vi "GetEdgeMenu.vi"(0 "reference":refnum<class "ClassRelationshipEdge.lvclass">, 5 "error in (no error)":errorcluster) -> (14 "reference out":refnum<class "ClassRelationshipEdge.lvclass">, 15 "MenuOptions":string[](array[string]), 19 "error out":errorcluster)   [LabVIEW 2020, in "ClassRelationshipEdge.lvclass"]
uses:
  <resource>/Framework/Providers/Open_GDS/UML/ClassRelationshipEdge_class/ClassRelationshipEdge.lvclass
  <resource>/Framework/Providers/Open_GDS/UML/SegmentedLineEdge_class/SegmentedLineEdge.lvclass
  <resource>/Framework/Providers/Open_GDS/UML/BentStyle_class/BentStyle.lvclass
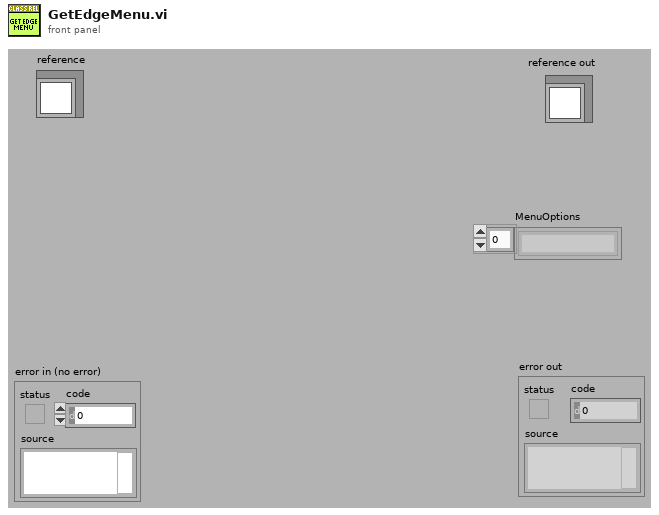
[diagram p1: front panel]
types:
  T1 = typedef "ClassRelationshipEdge.lvclass/ObjectAttributes.ctl" = cluster{"bentStyleRef":refnum<class "BentStyle.lvclass">, "startConnectionOffset":cluster{"x":i32, "y":i32}, "endConnectionOffset":cluster{"x":i32, "y":i32}, "MidLineOffset":cluster{"x":i32, "y":i32}, "DepClass":T2}
  T2 = typedef "ReversedEngineering_ViDependencyDetailsType.ctl" = cluster{"ThisVIs/Ctls":path[], "Dependent_VIs/Ctls":path[]}
  T3 = typedef "BentStyle.lvclass/BentStyleType.ctl" = enum16{"STRAIGHT", "HV", "VH", "HVH", "VHV", "ARC"}
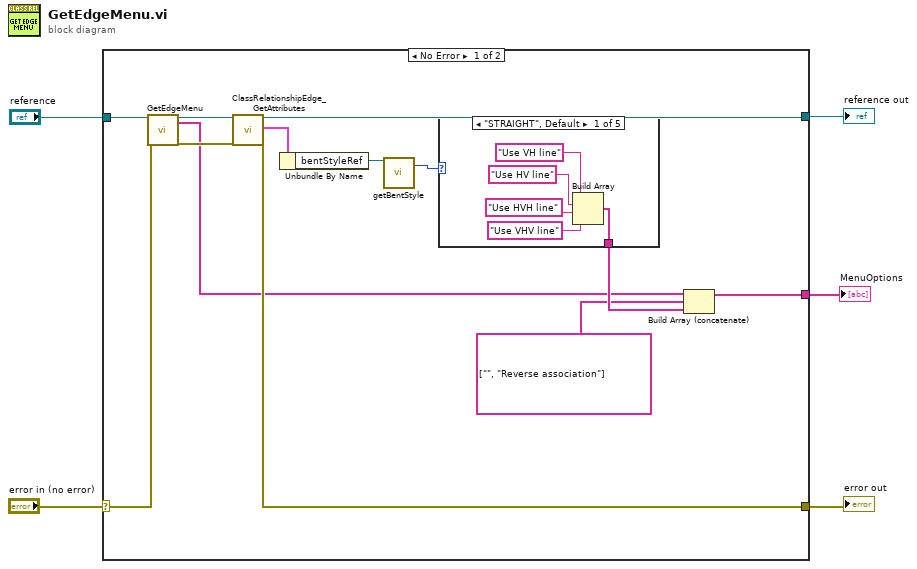
[diagram p0: block diagram]
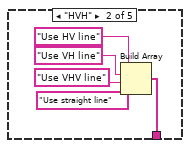
[diagram p2: hidden frame]
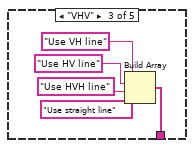
[diagram p3: hidden frame]
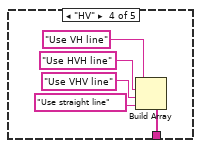
[diagram p4: hidden frame]
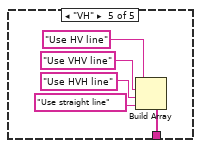
[diagram p5: hidden frame]
diagram:
  n1 = case shown="No Error" "error in (no error)" {
    selector: "error in (no error)" -> [w9 w44]
    tunnel: "reference" -> [w11 w45]
    tunnel: [w17 w44] -> w3
    tunnel: [w18 w45] -> w2
    tunnel: [w16 _] -> w1
    frame No Error {
      n2 = call-parent "GetEdgeMenu.vi"("reference"=w11, "error in (no error)"=w9) -> ("reference out"=w10:refnum<class "ClassRelationshipEdge.lvclass">, "MenuOptions"=w7:string[], "error out"=w8:errorcluster)  [unwired: 15 in]
      n3 = call <resource>:"ClassRelationshipEdge_GetAttributes.vi"("reference in"=w10, "error in (no error)"=w8) -> ("reference out"=w18:refnum<class "ClassRelationshipEdge.lvclass">, "Data"=w6:T1, "error out"=w17:errorcluster)  [unwired: 1 in, 14 out]
      n4 = Unbundle By Name(w6) -> ("bentStyleRef"=w15:refnum<class "BentStyle.lvclass">)
      n5 = call-dynamic "getBentStyle.vi"("reference"=w15) -> ("bentStyle"=w14:T3)  [unwired: 16 in, 2 out]
      n6 = case shown="\"STRAIGHT\", Default" w14 {
        tunnel: [w21 w26 w31 w37 w42] -> w13
        frame "STRAIGHT", Default {
          n7 = Build Array("Use VH line" ("String"), "Use HV line" ("String"), "Use HVH line" ("String"), "Use VHV line" ("String")) -> (w21:string[])
        }
        frame "HVH" {
          n8 = Build Array("Use HV line" ("String"), "Use VH line" ("String"), "Use VHV line" ("String"), "Use straight line" ("String")) -> (w26:string[])
        }
        frame "VHV" {
          n9 = Build Array("Use VH line" ("String"), "Use HV line" ("String"), "Use HVH line" ("String"), "Use straight line" ("String")) -> (w31:string[])
        }
        frame "HV" {
          n10 = Build Array("Use VH line" ("String"), "Use HVH line" ("String"), "Use VHV line" ("String"), "Use straight line" ("String")) -> (w37:string[])
        }
        frame "VH" {
          n11 = Build Array("Use HV line" ("String"), "Use VHV line" ("String"), "Use HVH line" ("String"), "Use straight line" ("String")) -> (w42:string[])
        }
      }
      n12 = Build Array (concatenate)(w7, string[] ["", "Reverse association"] ("array"), w13) -> (w16:string[])
    }
    frame Error {
    }
  }
  "reference out" <- w2
  "error out" <- w3
  "MenuOptions" <- w1
